vi "libssh2_knownhost_free.vi"(8 "error in (no error)":errorcluster, 11 "known hosts":T1) -> (0 "error out":errorcluster)   [LabVIEW 2013, in "libssh2.lvlib"]
doc: "Frees a collection of known hosts."
uses:
  libssh2.lvlib
  Known Hosts Refnum.ctl
  libssh2.dll
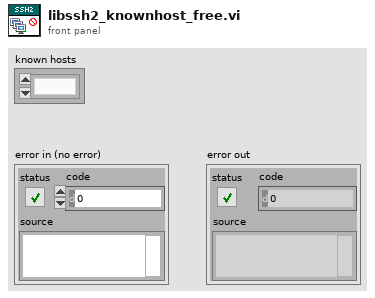
[diagram p1: front panel]
types:
  T1 = typedef "libssh2.lvlib/Known Hosts Refnum.ctl" = refnum<k1>
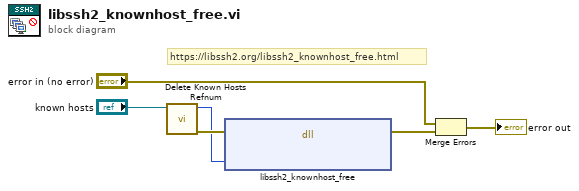
[diagram p0: block diagram]
diagram:
  # "https://libssh2.org/libssh2_knownhost_free.html"
  n1 = call "Delete Known Hosts Refnum.vi"("known hosts"="known hosts") -> ("error out"=w5:errorcluster, "LIBSSH2_KNOWNHOSTS*"=w3:u64)  [unwired: 9 in]
  n2 = dll-call lib="C:/Users/pasca/source/repos/libssh2-labview/libssh2**.*" fn="libssh2_knownhost_free"(error in=w5, "hosts"=w3) -> (error out=w6:errorcluster)  [unwired: 4 in, 1 out]
  n3 = Merge Errors("error in (no error)", w6) -> (→"error out":errorcluster)
